vi "FdxCmdTxQueueStatusCvi.vi"(8 "error in":errorcluster, 11 "InstrumentHandle":u32) -> (0 "error out":errorcluster, 1 "TxQueueStatus":T1 {"QueueStatus" items=["FDX_QUE_EMPTY", "FDX_QUE_FILLED", "FDX_QUE_FULL", "FDX_QUE_SENT", "FDX_QUE_CYCL_RUN", "FDX_QUE_CYCL_SENT"]}, 3 "InstrumentHandle":u32)   [LabVIEW 2020, in "AIM664LV.lvlib"]
doc: "This function is used to retrieve the AFDX Transmit Queue status when in Generic or Replay Transmit Mode."
uses:
  AIM664LV.lvlib
  AFDX_LibraryAdmin/FdxGlobalDllPath.vi
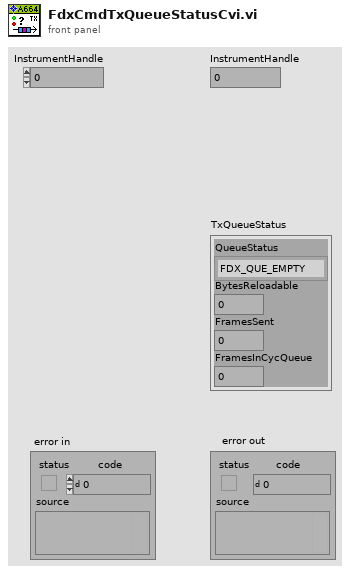
[diagram p1: front panel]
types:
  T1 = cluster{"QueueStatus":i32, "BytesReloadable":u32, "FramesSent":u32, "FramesInCycQueue":u32}
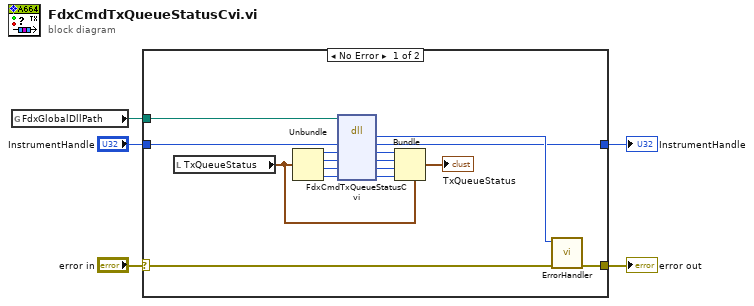
[diagram p0: block diagram]
diagram:
  n1 = global read "FdxGlobalDllPath.vi" "FdxGlobalDllPath"() -> (w3:path)
  n2 = case shown="No Error" "error in" {
    selector: "error in" -> [w20 w23]
    tunnel: [w21 w23] -> w5
    tunnel: w3 -> [w8 _]
    tunnel: "InstrumentHandle" -> [w7 w22]
    tunnel: [w6 w22] -> w1
    frame No Error {
      n3 = local read "TxQueueStatus"() -> (w13:T1)
      n4 = Unbundle(w13) -> ("QueueStatus"=w12:i32, "BytesReloadable"=w11:u32, "FramesSent"=w10:u32, "FramesInCycQueue"=w9:u32)
      n5 = dll-call lib="aim_fdx.19.dll" fn="FdxCmdTxQueueStatusCvi"(path in=w8, "InstrumentHandle"=w7, "QueueStatus"=w12, "BytesReloadable"=w11, "FramesSent"=w10, "FramesInCycQueue"=w9) -> ("status"=w19:i32, "InstrumentHandle"=w6:u32, "QueueStatus"=w18:i32, "BytesReloadable"=w17:u32, "FramesSent"=w16:u32, "FramesInCycQueue"=w15:u32)  [unwired: 2 in, 2 out]
      n6 = Bundle(cluster=w13, "QueueStatus"=w18, "BytesReloadable"=w17, "FramesSent"=w16, "FramesInCycQueue"=w15) -> (→"TxQueueStatus":T1)
      n7 = call "ErrorHandler.vi"("error in"=w20, "AIM Error"=w19) -> ("error out"=w21:errorcluster)  [unwired: 9 in]
    }
    frame Error {
    }
  }
  "error out" <- w5
  "InstrumentHandle" <- w1
